vi "find channels.vi"(11 "Cluster in":T1) -> (3 "Cluster out":T1)   [LabVIEW 2018]
uses:
  custom sub vis/speedlineData.ctl
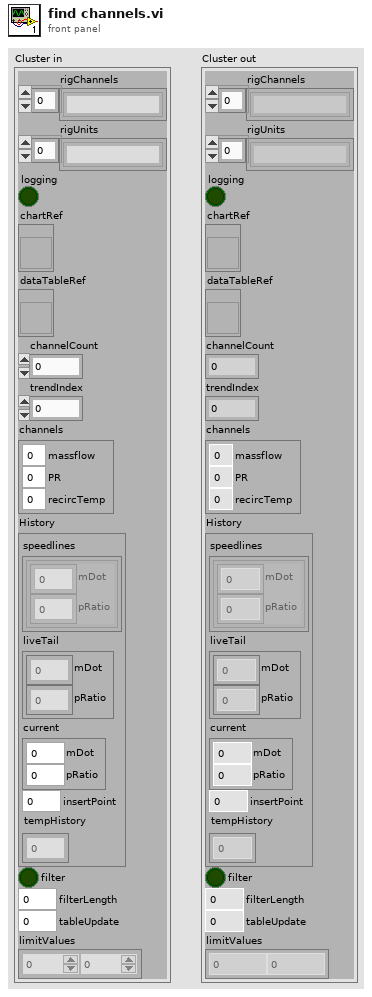
[diagram p1: front panel]
types:
  T1 = typedef "speedlineData.ctl" = cluster{"rigChannels":string[], "rigUnits":string[], "logging":bool, "chartRef":refnum<vi>, "dataTableRef":refnum<vi>, "channelCount":i32, "trendIndex":i32, "channels":cluster{"massflow":i32, "PR":i32, "recircTemp":i32}, "History":cluster{"speedlines":cluster{"mDot":dbl[], "pRatio":dbl[]}[], "liveTail":cluster{"mDot":dbl[], "pRatio":dbl[]}, "current":cluster{"mDot":dbl, "pRatio":dbl}, "insertPoint":i32, "tempHistory":dbl[][]}, "filter":bool, "filterLength":i32, "tableUpdate":i16, "limitValues":dbl[][]}
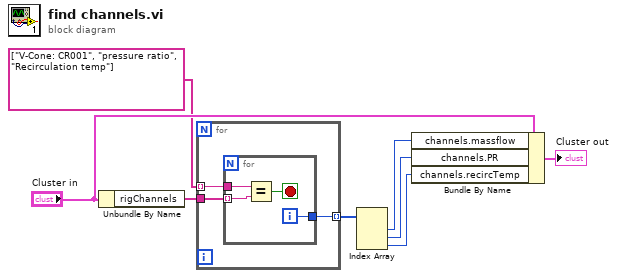
[diagram p0: block diagram]
diagram:
  n1 = Unbundle By Name("Cluster in") -> ("rigChannels"=w5:string[])
  n2 = for {
    tunnel: string[] ["V-Cone: CR001", "pressure ratio", "Recirculation temp"] -> [w11] mode=indexing
    tunnel: w5 -> [w10]
    tunnel: [w9] -> w4 mode=indexing
    n3 = for {
      tunnel: w11 -> [w15]
      tunnel: w10 -> [w14] mode=indexing
      tunnel: [w12] -> w9
      i -> [w12]
      stop <- w13 stop-if-true
      n4 = Equal?(x=w15, y=w14) -> (x = y?=w13:bool)
    }
  }
  n5 = Index Array(array=w4) -> (element #1=w3:i32, element #2=w2:i32, element #3=w1:i32)  [unwired: 3 in]
  n6 = Bundle By Name(cluster="Cluster in", "channels.massflow"=w3, "channels.PR"=w2, "channels.recircTemp"=w1) -> (→"Cluster out":T1)
